vi "LJM logger get user directory.vi"() -> (3 "User Directory":path)   [LabVIEW 2026]
uses:
  <vilib>/registry/registry.llb/Registry RtKey.ctl
  <vilib>/registry/registry.llb/Read Registry Value Simple STR.vi
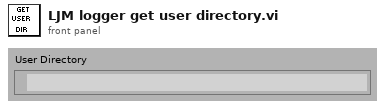
[diagram p1: front panel]
types:
  T1 = typedef "Registry RtKey.ctl" = enum32{"HKEY_CLASSES_ROOT", "HKEY_CURRENT_USER", "HKEY_LOCAL_MACHINE", "HKEY_USERS", "HKEY_PERFORMANCE_DATA", "HKEY_CURRENT_CONFIG", "HKEY_DYN_DATA"}
  T2 = typedef "Registry refnum.ctl" = refnum<k1>
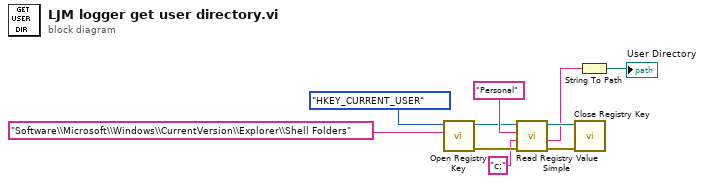
[diagram p0: block diagram]
diagram:
  n1 = call <vilib>:"Open Registry Key.vi"("subkey"="Software\\Microsoft\\Windows\\CurrentVersion\\Explorer\\Shell Folders", "root key (HKEY_LOCAL_MACHINE)"=Registry_RtKey."HKEY_CURRENT_USER") -> ("error out"=w8:errorcluster, "refnum out"=w5:T2)  [unwired: 8 in]
  n2 = call-poly <vilib>:"Read Registry Value Simple.vi"("error in (no error)"=w8, "default data"="c:", "value"="Personal", "refnum"=w5) -> ("error out"=w3:errorcluster, "String/Binary data"=w2:string, "refnum out"=w4:T2)  [unwired: 2 in, 1 out]
  n3 = call <vilib>:"Close Registry Key.vi"("error in (no error)"=w3, "refnum"=w4) -> ()  [unwired: 5 in, 1 out]
  n4 = String To Path(string=w2) -> (path=→"User Directory":path)
